vi "GetDiagramUID.vi"(6 "error in":errorcluster, 9 "FlatSequenceFrame in":refnum<class "FlatSequenceFrame.lvclass">) -> (0 "error out":errorcluster, 3 "FlatSequenceFrame out":refnum<class "FlatSequenceFrame.lvclass">, 4 "Diagram.UID":i32)   [LabVIEW 2014, in "FlatSequenceFrame.lvclass"]
uses:
  FlatSequenceFrame.lvclass
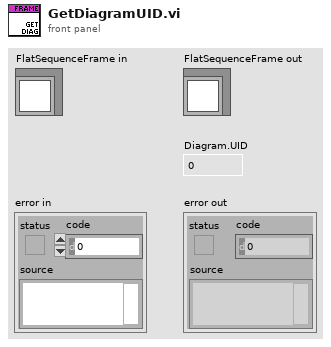
[diagram p1: front panel]
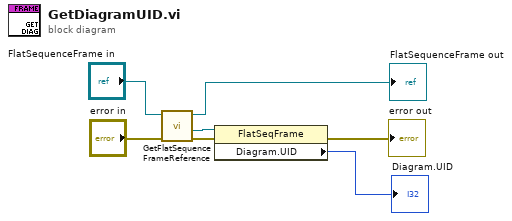
[diagram p0: block diagram]
diagram:
  n1 = call "GetFlatSequenceFrameReference.vi"("error in"="error in", "FlatSequence in"="FlatSequenceFrame in") -> ("error out"=w3:errorcluster, "reference out"=w4:refnum<vi>, "FlatSequence out"=→"FlatSequenceFrame out":refnum<class "FlatSequenceFrame.lvclass">)  [unwired: 7 in]
  n2 = property class="FlatSeqFrame"(reference=w4, error in=w3) -> (error out=→"error out":errorcluster, "Diagram.UID"=→"Diagram.UID":i32)  [unwired: 1 out]
